vi "KE24xx, Current Leakage Setup.vi"(8 "error in":errorcluster, 9 "Source Level (0.0 V)":dbl[unit] format="%.3f", 10 "Compliance Level (10 mV)":dbl[unit]=0.01 format="%.3f", 11 "VISA resource name":refnum<visa-resource-name>="GPIB0::9::INSTR") -> (0 "error out":errorcluster, 3 "VISA resource dup":refnum<visa-resource-name>)   [LabVIEW 2010]
uses:
  <instrlib>/Keithley 24XX/Keithley 24XX.lvlib
panel:
  in  "Initial Range (10 mA)":dbl[unit]=0.01 format="%.3f"
  in  "Function (1: Current)":u16(ring)=1 items=["Volts", "Current", "Resistance"]
  in  "Autorange (F)":bool
  # "Final Range = Initial Range / 100.0"
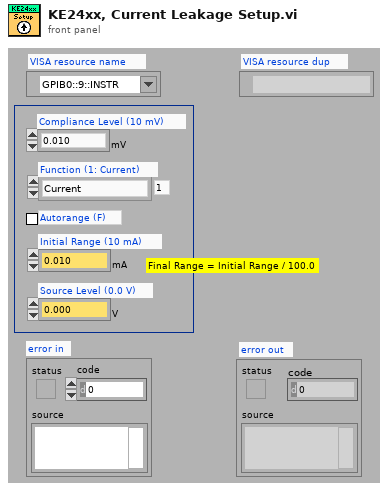
[diagram p1: front panel]
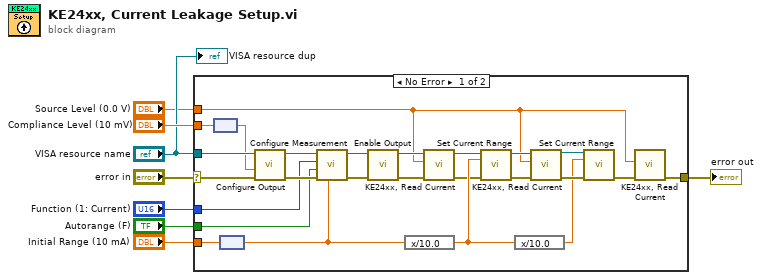
[diagram p0: block diagram]
diagram:
  n1 = case shown="No Error" "error in" {
    selector: "error in" -> [w32 w34]
    tunnel: [w16 w34] -> w8
    tunnel: "Compliance Level (10 mV)" -> [w33 _]
    tunnel: "VISA resource name" -> [w28 _]
    tunnel: "Autorange (F)" -> [w25 _]
    tunnel: "Function (1: Current)" -> [w26 _]
    tunnel: "Initial Range (10 mA)" -> [w24 _]
    tunnel: "Source Level (0.0 V)" -> [w12 _]
    frame No Error {
      n2 = node(w33) -> (w11:dbl)
      n3 = node(w24) -> (w23:dbl)
      n4 = call <instrlib>:"Configure Output.vi"("error in (no error)"=w32, "Compliance  Level (0.1)"=w11, "VISA resource name"=w28) -> ("error out"=w31:errorcluster, "VISA resource name out"=w29:refnum<visa-resource-name>)  [unwired: 7 in]
      n5 = call <instrlib>:"Configure Measurement.vi"("Manual Range (1.0)"=w23, "error in (no error)"=w31, "Enable Auto Range (T:Enable)"=w25, "Function (0: Volts)"=w26, "VISA resource name"=w29) -> ("error out"=w30:errorcluster, "VISA resource name out"=w27:refnum<visa-resource-name>)  [unwired: 5 in]
      n6 = call <instrlib>:"Enable Output.vi"("error in (no error)"=w30, "VISA resource name"=w27) -> ("error out"=w22:errorcluster, "VISA resource name out"=w13:refnum<visa-resource-name>)  [unwired: 8 in]
      n7 = expression code="x/10.0"(w23) -> (w21:dbl)
      n8 = call "KE24xx, Read Current.vi"("error in"=w22, "Source Level (0.0 V)"=w12, "VISA resource name"=w13) -> ("error out"=w10:errorcluster, "VISA resource dup"=w9:refnum<visa-resource-name>)  [unwired: 6 in, 1 out]
      n9 = call "Set Current Range.vi"("VISA resource name"=w9, "Range"=w21, "error in (no error)"=w10) -> ("VISA resource name out"=w14:refnum<visa-resource-name>, "error out"=w19:errorcluster)  [unwired: 11 in]
      n10 = expression code="x/10.0"(w21) -> (w18:dbl)
      n11 = call "KE24xx, Read Current.vi"("error in"=w19, "Source Level (0.0 V)"=w12, "VISA resource name"=w14) -> ("error out"=w20:errorcluster, "VISA resource dup"=w15:refnum<visa-resource-name>)  [unwired: 6 in, 1 out]
      n12 = call "Set Current Range.vi"("VISA resource name"=w15, "Range"=w18, "error in (no error)"=w20) -> ("error out"=w17:errorcluster)  [unwired: 11 in, 1 out]
      n13 = call "KE24xx, Read Current.vi"("error in"=w17, "Source Level (0.0 V)"=w12) -> ("error out"=w16:errorcluster)  [unwired: 7 in, 2 out]
    }
    frame Error {
    }
  }
  "error out" <- w8
  "VISA resource dup" <- "VISA resource name"
